vi "ZhiYuan ZDS Series for TCP Acquire Waveform Continuously.vi"() -> ()   [LabVIEW 2015]
doc: "This example shows how to use autosetup and acquire a waveform continuously on a single channel.\n\n<B>Note:</B> In this example, each record is acquired independently and not as a continuous stream of data."
uses:
  ZhiYuan ZDS Series for TCP.lvlib
  Public/Data/Read Waveform (Single).vi
panel:
  in  "Maximum Time (ms)":u32=5000
  in  "stop":bool
  out "Waveform Data":dbl[](graph)
  in  "Channel":u16(ring)=1 items=["Channel 1"=1, "Channel 2"=2, "Channel 3"=3, "Channel 4"=4]
  in  "VISA resource name":refnum<visa-resource-name>
  # "(c) 2012 National Instruments.  ALL RIGHTS RESERVED."
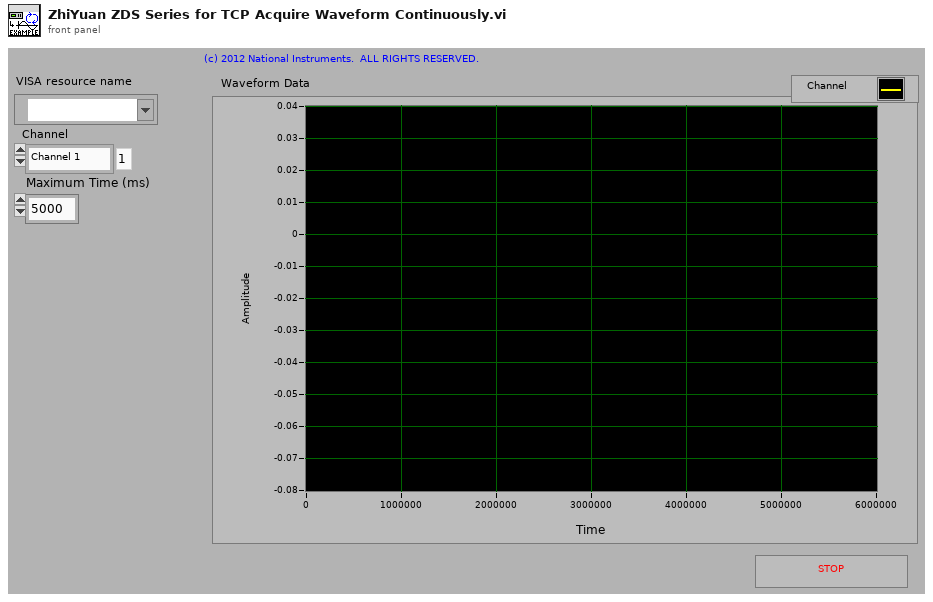
[diagram p1: front panel]
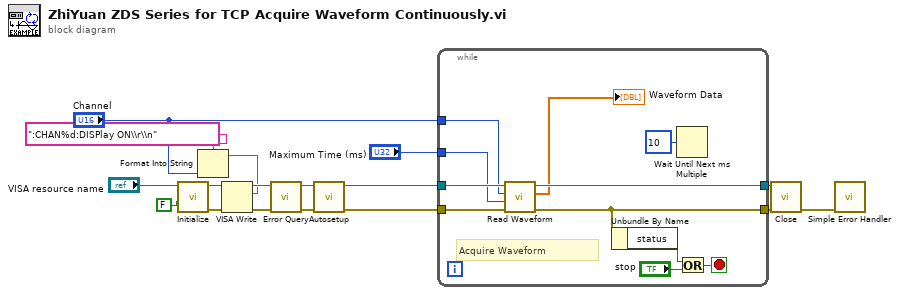
[diagram p0: block diagram]
diagram:
  n1 = call "Initialize.vi"("Reset (True)"=FALSE, "VISA resource name"="VISA resource name") -> ("error out"=w7:errorcluster, "VISA resource name out"=w8:refnum<visa-resource-name>)  [unwired: 8 in]
  n2 = Format Into String(format string=":CHAN%d:DISPlay ON\\r\\n", "Channel") -> (resulting string=w3:string)  [unwired: 2 in, 1 out]
  n3 = VISA Write(VISA resource name=w8, write buffer=w3, error in (no error)=w7) -> (VISA resource name out=w9:refnum<visa-resource-name>, error out=w10:errorcluster)  [unwired: 1 out]
  n4 = call "Error Query.vi"("error in (no error)"=w10, "VISA resource name"=w9) -> ("error out"=w5:errorcluster, "VISA resource name out"=w6:refnum<visa-resource-name>)  [unwired: 6 in, 2 out]
  n5 = call "Autosetup.vi"("error in (no error)"=w5, "VISA resource name"=w6) -> ("error out"=w12:errorcluster, "VISA resource name out"=w13:refnum<visa-resource-name>)  [unwired: 8 in]
  n6 = while {
    tunnel: w13 -> [w24]
    tunnel: w12 -> [w20]
    tunnel: [w23] -> w16
    tunnel: [w19] -> w15
    tunnel: "Channel" -> [w21]
    tunnel: "Maximum Time (ms)" -> [w22]
    stop <- w27 stop-if-true
    # "Acquire Waveform"
    n7 = call-poly "Read Waveform.vi"("error in (no error)"=w20, "Maximum Time (5000 ms)"=w22, "Channel (1: Channel 1)"=w21, "VISA resource name"=w24) -> ("error out"=w19:errorcluster, "Waveform Data"=→"Waveform Data":dbl[], "VISA resource name out"=w23:refnum<visa-resource-name>)  [unwired: 5 in]
    n8 = Unbundle By Name(w19) -> ("status"=w26:bool)
    n9 = Wait Until Next ms Multiple(millisecond multiple=u32 10) -> ()  [unwired: 1 out]
    n10 = Or(x=w26, y="stop") -> (x .or. y?=w27:bool)
  }
  n11 = call "Close.vi"("error in (no error)"=w15, "VISA resource name"=w16) -> ("error out"=w17:errorcluster)  [unwired: 9 in]
  n12 = call <vilib>:"Simple Error Handler.vi"("error in (no error)"=w17) -> ()  [unwired: 4 in, 5 out]
